vi "SSL Referee Stage to GUI Stage.vi"(11 "stage":u64) -> (3 "String":string)   [LabVIEW 2016]
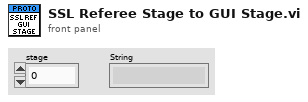
[diagram p1: front panel]
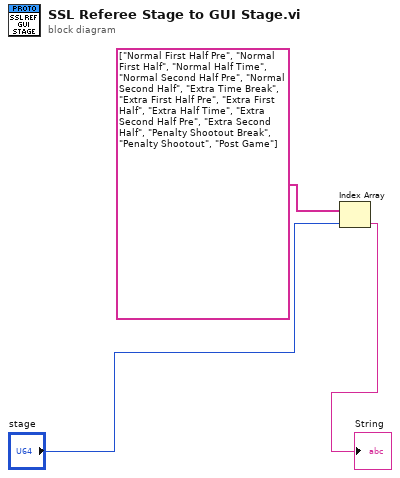
[diagram p0: block diagram]
diagram:
  n1 = Index Array(array=string[] ["Normal First Half Pre", "Normal First Half", "Normal Half Time", "Normal Second Half Pre", "Normal Second Half", "Extra Time Break", "Extra First Half Pre", "Extra First Half", "Extra Half Time", "Extra Second Half Pre", "Extra Second Half", "Penalty Shootout Break", "Penalty Shootout", "Post Game"], index="stage") -> (element=→"String":string)
